vi "Configuration Editor.vi"() -> ()   [LabVIEW 2012]
uses:
  Devices/Alicat/Configuration/Controller Config.ctl
  Controls/pasLasCtl.ctl
  Utilities/FPGA/Controls/FPGAConfig.ctl
  Reusable/PAS/Main/Controls/Laser Modulation.ctl
  Controls/pasCellTEC.ctl
  Controls/pasTECen.ctl
  Devices/Alicat/Alicat.lvlib
panel:
  in  "Tab Control":enum32{"General", "CRD", "PAS"}(tab)
  in  "valveCfg":T1
  in  "MFC COM":refnum<visa-resource-name> caption="Alicat Bank COM"
  in  "System Cluster":T2
  in  "temp":cluster{"hum":sgl, "dry":sgl} caption="Temperatures (degC)" {"dry" format="%#.2f"; "hum" format="%#.2f"}
  in  "CRDLaserCfg":cluster{"f (Hz)":dbl, "Duty Cycle (%)":dbl} caption="Laser Parameters"
  in  "CRD MFC":T3[](array[typedef]) caption="MFC Config"
  in  "mTECCfg":T4 caption="Main TEC"
  in  "PAS_TEC_Cfg":cluster{"pasTcell":T5, "pasTECEn":T6} caption="Cell TECs"
  in  "pasLasCtl":T7={"Laser Output"={"Span"={"ch 1"=1.5, "ch 2"=1.5, "ch 3"=5.0, "ch 4"=5.0, "ch 5"=5.0}, "mod"={"ch 1"=enum."Sine", "ch 2"=enum."Sine", "ch 3"=enum."Sine", "ch 4"=enum."Sine", "ch 5"=enum."Sine"}}, "f0"={"Cell 1"=1360.2863, "Cell 2"=1358.2849, "Cell 3"=1355.6958, "Cell 4"=1355.4038, "Cell 5"=1352.1854}, "drive"=FALSE, "lasSysPow"=TRUE, "Speake Voltage"=0.0} caption="Laser Control" {"Laser Output"."Span"."ch 5" min=0 max=20; "Laser Output"."Span"."ch 4" min=0 max=20; "Laser Output"."Span"."ch 3" min=0 max=20; "Laser Output"."Span"."ch 2" min=0 max=20; "Laser Output"."Span"."ch 1" min=0 max=20; "f0"."Cell 1" min=0 max=2000 step=1 format="%#.2f"; "f0"."Cell 2" min=0 max=2000 step=1 format="%#.2f"; "f0"."Cell 3" min=0 max=2000 step=1 format="%#.2f"; "f0"."Cell 4" min=0 max=2000 step=1 format="%#.2f"; "f0"."Cell 5" min=0 max=2000 step=1 format="%#.2f"}
  in  "PAS MFC":T3[](array[typedef]) caption="Alicat Controllers"
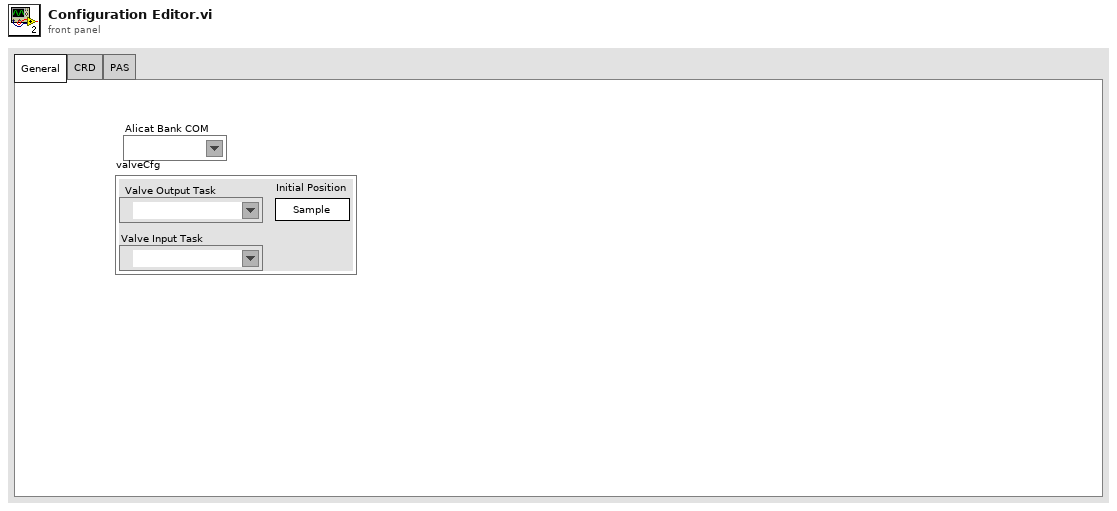
[diagram p1: front panel]
types:
  T1 = cluster{"valveIn":refnum<k21>, "valveOut":refnum<k21>, "valvePos":bool}
  T2 = cluster{"enable":cluster{"med":bool, "high":bool}}
  T3 = typedef "Alicat.lvlib/Controller Config.ctl" = cluster{"Name":string, "Address":string, "Q0":sgl}
  T4 = cluster{"COM":refnum<visa-resource-name>, "Setpoint":dbl}
  T5 = typedef "pasCellTEC.ctl" = cluster{"Cell 1":sgl, "Cell 2":sgl, "Cell 3":sgl, "Cell 4":sgl, "Cell 5":sgl}
  T6 = typedef "pasTECen.ctl" = cluster{"Cell 1":bool, "Cell 2":bool, "Cell 3":bool, "Cell 4":bool, "Cell 5":bool}
  T7 = typedef "pasLasCtl.ctl" = cluster{"Laser Output":T8, "f0":cluster{"Cell 1":sgl, "Cell 2":sgl, "Cell 3":sgl, "Cell 4":sgl, "Cell 5":sgl}, "drive":bool, "lasSysPow":bool, "Speake Voltage":dbl}
  T8 = typedef "FPGAConfig.ctl" = cluster{"Span":cluster{"ch 1":sgl, "ch 2":sgl, "ch 3":sgl, "ch 4":sgl, "ch 5":sgl}, "mod":cluster{"ch 1":T9, "ch 2":T9, "ch 3":T9, "ch 4":T9, "ch 5":T9}}
  T9 = typedef "Laser Modulation.ctl" = enum8{"Sine", "Square"}
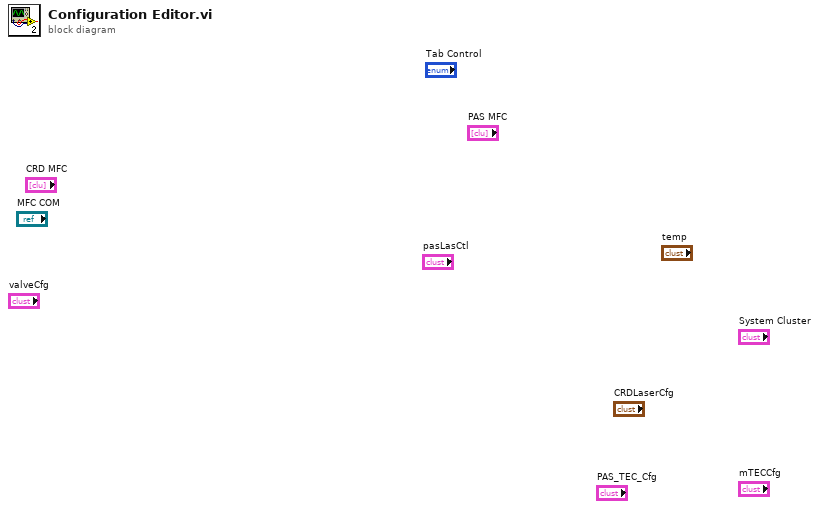
[diagram p0: block diagram]
diagram:
